vi "Translate ActiveX errors.vi"(8 "error in (no error)":errorcluster, 10 "ActiveX return":i32, 11 "AOTF in":refnum<class "AOTF.lvclass">) -> (0 "error out":errorcluster, 3 "AOTF out":refnum<class "AOTF.lvclass">)   [LabVIEW 2012, in "AOTF.lvclass"]
uses:
  AOTF.lvclass
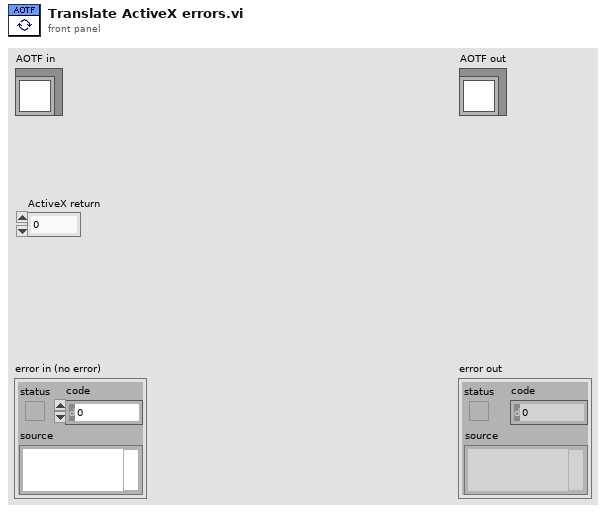
[diagram p1: front panel]
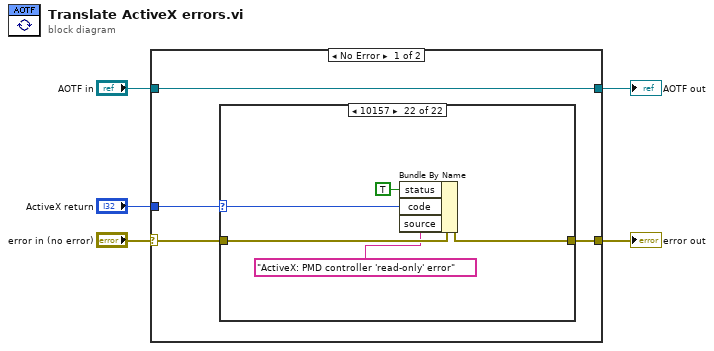
[diagram p0: block diagram]
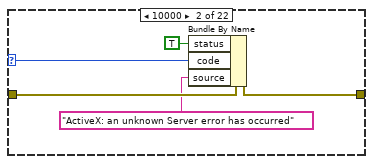
[diagram p3: hidden frame]
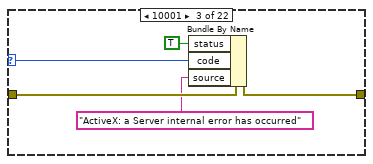
[diagram p4: hidden frame]
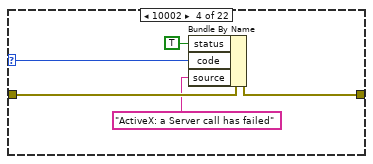
[diagram p5: hidden frame]
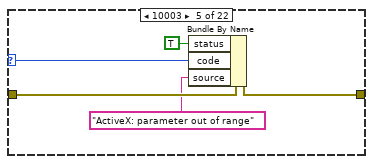
[diagram p6: hidden frame]
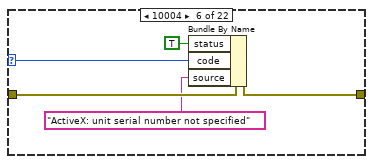
[diagram p7: hidden frame]
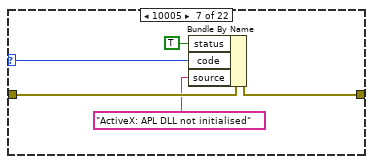
[diagram p8: hidden frame]
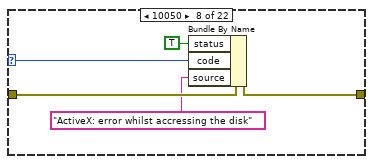
[diagram p9: hidden frame]
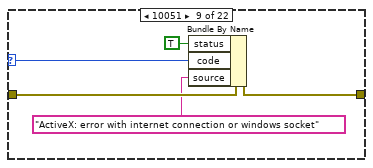
[diagram p10: hidden frame]
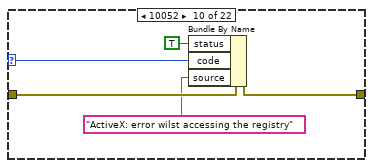
[diagram p11: hidden frame]
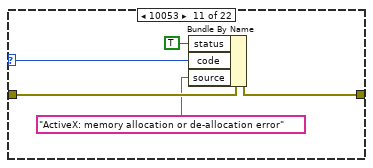
[diagram p12: hidden frame]
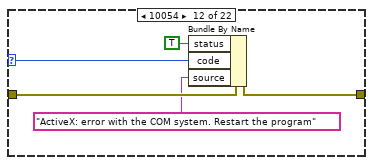
[diagram p13: hidden frame]
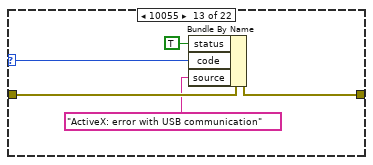
[diagram p14: hidden frame]
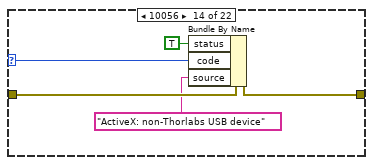
[diagram p15: hidden frame]
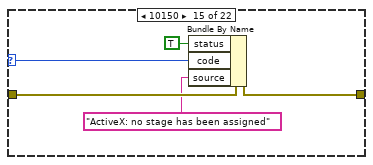
[diagram p16: hidden frame]
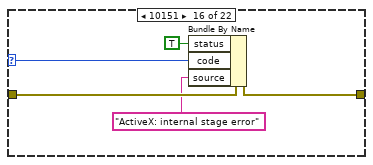
[diagram p17: hidden frame]
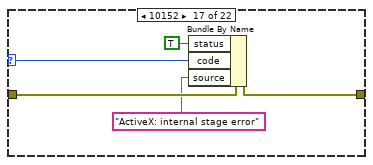
[diagram p18: hidden frame]
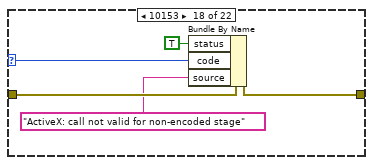
[diagram p19: hidden frame]
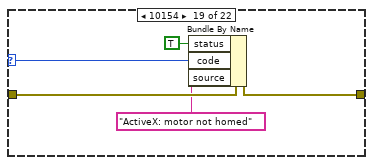
[diagram p20: hidden frame]
diagram:
  n1 = case shown="No Error" "error in (no error)" {
    selector: "error in (no error)" -> [w8 w117]
    tunnel: [w7 w117] -> w4
    tunnel: [w9 w116] -> w2
    tunnel: "AOTF in" -> [w9 w116]
    tunnel: "ActiveX return" -> [w6 _]
    frame No Error {
      n2 = case shown="10157" w6 {
        selector: w6 -> [_ w13 w18 w23 w28 w33 w38 w43 w48 w53 w58 w63 w68 w73 w78 w83 w88 w93 w98 w103 w108 w113]
        tunnel: w8 -> [w10 w15 w20 w25 w30 w35 w40 w45 w50 w55 w60 w65 w70 w75 w80 w85 w90 w95 w100 w105 w110 w115]
        tunnel: [w10 w14 w19 w24 w29 w34 w39 w44 w49 w54 w59 w64 w69 w74 w79 w84 w89 w94 w99 w104 w109 w114] -> w7
        frame 0, Default {
        }
        frame 10000 {
          n3 = Bundle By Name(cluster=w15, "status"=TRUE, "code"=w13, "source"="ActiveX: an unknown Server error has occurred") -> (w14:errorcluster)
        }
        frame 10001 {
          n4 = Bundle By Name(cluster=w20, "status"=TRUE, "code"=w18, "source"="ActiveX: a Server internal error has occurred") -> (w19:errorcluster)
        }
        frame 10002 {
          n5 = Bundle By Name(cluster=w25, "status"=TRUE, "code"=w23, "source"="ActiveX: a Server call has failed") -> (w24:errorcluster)
        }
        frame 10003 {
          n6 = Bundle By Name(cluster=w30, "status"=TRUE, "code"=w28, "source"="ActiveX: parameter out of range") -> (w29:errorcluster)
        }
        frame 10004 {
          n7 = Bundle By Name(cluster=w35, "status"=TRUE, "code"=w33, "source"="ActiveX: unit serial number not specified") -> (w34:errorcluster)
        }
        frame 10005 {
          n8 = Bundle By Name(cluster=w40, "status"=TRUE, "code"=w38, "source"="ActiveX: APL DLL not initialised") -> (w39:errorcluster)
        }
        frame 10050 {
          n9 = Bundle By Name(cluster=w45, "status"=TRUE, "code"=w43, "source"="ActiveX: error whilst accressing the disk") -> (w44:errorcluster)
        }
        frame 10051 {
          n10 = Bundle By Name(cluster=w50, "status"=TRUE, "code"=w48, "source"="ActiveX: error with internet connection or windows socket") -> (w49:errorcluster)
        }
        frame 10052 {
          n11 = Bundle By Name(cluster=w55, "status"=TRUE, "code"=w53, "source"="ActiveX: error wilst accessing the registry") -> (w54:errorcluster)
        }
        frame 10053 {
          n12 = Bundle By Name(cluster=w60, "status"=TRUE, "code"=w58, "source"="ActiveX: memory allocation or de-allocation error") -> (w59:errorcluster)
        }
        frame 10054 {
          n13 = Bundle By Name(cluster=w65, "status"=TRUE, "code"=w63, "source"="ActiveX: error with the COM system. Restart the program") -> (w64:errorcluster)
        }
        frame 10055 {
          n14 = Bundle By Name(cluster=w70, "status"=TRUE, "code"=w68, "source"="ActiveX: error with USB communication") -> (w69:errorcluster)
        }
        frame 10056 {
          n15 = Bundle By Name(cluster=w75, "status"=TRUE, "code"=w73, "source"="ActiveX: non-Thorlabs USB device") -> (w74:errorcluster)
        }
        frame 10150 {
          n16 = Bundle By Name(cluster=w80, "status"=TRUE, "code"=w78, "source"="ActiveX: no stage has been assigned") -> (w79:errorcluster)
        }
        frame 10151 {
          n17 = Bundle By Name(cluster=w85, "status"=TRUE, "code"=w83, "source"="ActiveX: internal stage error") -> (w84:errorcluster)
        }
        frame 10152 {
          n18 = Bundle By Name(cluster=w90, "status"=TRUE, "code"=w88, "source"="ActiveX: internal stage error") -> (w89:errorcluster)
        }
        frame 10153 {
          n19 = Bundle By Name(cluster=w95, "status"=TRUE, "code"=w93, "source"="ActiveX: call not valid for non-encoded stage") -> (w94:errorcluster)
        }
        frame 10154 {
          n20 = Bundle By Name(cluster=w100, "status"=TRUE, "code"=w98, "source"="ActiveX: motor not homed") -> (w99:errorcluster)
        }
        frame 10155 {
          n21 = Bundle By Name(cluster=w105, "status"=TRUE, "code"=w103, "source"="ActiveX: motor disabled") -> (w104:errorcluster)
        }
        frame 10156 {
          n22 = Bundle By Name(cluster=w110, "status"=TRUE, "code"=w108, "source"="ActiveX: PMD processor message error") -> (w109:errorcluster)
        }
        frame 10157 {
          n23 = Bundle By Name(cluster=w115, "status"=TRUE, "code"=w113, "source"="ActiveX: PMD controller 'read-only' error") -> (w114:errorcluster)
        }
      }
    }
    frame Error {
    }
  }
  "error out" <- w4
  "AOTF out" <- w2
